vi "FCGI request worker.vi"(11 "exec queue":refnum<queue>) -> ()   [LabVIEW 2013]
uses:
  worker package.ctl
  application request.ctl
  FCGI begin request role.ctl
  default responder action.vi
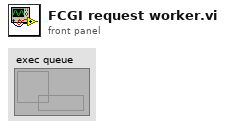
[diagram p1: front panel]
types:
  T1 = typedef "worker package.ctl" = cluster{"TCP Connection":refnum<k5>, "application request":T2}
  T2 = typedef "application request.ctl" = cluster{"request id":u16, "role":T3, "standard input":string, "data":string, "dictionary":variant, "close after response":bool}
  T3 = typedef "FCGI begin request role.ctl" = enum16{"none", "Responder", "Authorizer", "Filter"}
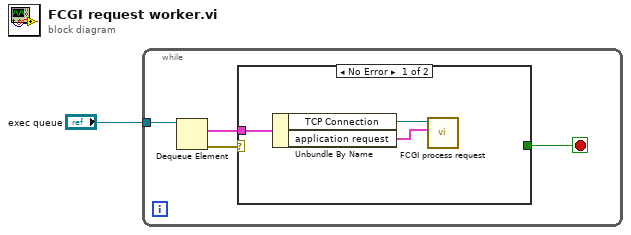
[diagram p0: block diagram]
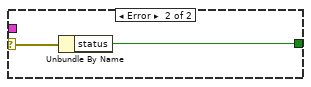
[diagram p2: hidden frame]
diagram:
  n1 = while {
    tunnel: "exec queue" -> [w5]
    stop <- w3 stop-if-true
    n2 = Dequeue Element(queue=w5) -> (element=w2:T1, error out=w4:errorcluster)  [unwired: 2 in, 2 out]
    n3 = case shown="No Error" w4 {
      selector: w4 -> [_ w10]
      tunnel: [_ w9] -> w3
      tunnel: w2 -> [w8 _]
      frame No Error {
        n4 = Unbundle By Name(w8) -> ("TCP Connection"=w7:refnum<k5>, "application request"=w6:T2)
        n5 = call "FCGI process request.vi"("application request"=w6, "connection"=w7) -> ()  [unwired: 10 in]
      }
      frame Error {
        n6 = Unbundle By Name(w10) -> ("status"=w9:bool)
      }
    }
  }
